vi "dfd_FXP_Expand Filter Quantizers.vi"(11 "FXPOPs":T1[](array[typedef]) {"source" items=["Coef a/k"=0, "Coef b/v"=7, "Input"=1, "Output"=2, "Multiplicand"=3, "Product"=4, "Sum"=5, "Delay"=6, "Gain"=8]}) -> (0 "Delay":T1={"source"=0, "is floating?"=FALSE, "o-mode"=enum."Wrap", "q-mode"=enum."Nearest", "wl"=1, "high limit"=0, "low limit"=0, "iwl"=0, "sign?"=TRUE} {"source" items=["Coef a/k"=0, "Coef b/v"=7, "Input"=1, "Output"=2, "Multiplicand"=3, "Product"=4, "Sum"=5, "Delay"=6, "Gain"=8]}, 1 "Sum":T1={"source"=0, "is floating?"=FALSE, "o-mode"=enum."Wrap", "q-mode"=enum."Nearest", "wl"=1, "high limit"=0, "low limit"=0, "iwl"=0, "sign?"=TRUE} {"source" items=["Coef a/k"=0, "Coef b/v"=7, "Input"=1, "Output"=2, "Multiplicand"=3, "Product"=4, "Sum"=5, "Delay"=6, "Gain"=8]}, 2 "Product":T1={"source"=0, "is floating?"=FALSE, "o-mode"=enum."Wrap", "q-mode"=enum."Nearest", "wl"=1, "high limit"=0, "low limit"=0, "iwl"=0, "sign?"=TRUE} {"source" items=["Coef a/k"=0, "Coef b/v"=7, "Input"=1, "Output"=2, "Multiplicand"=3, "Product"=4, "Sum"=5, "Delay"=6, "Gain"=8]}, 3 "Multiplicand":T1={"source"=0, "is floating?"=FALSE, "o-mode"=enum."Wrap", "q-mode"=enum."Nearest", "wl"=1, "high limit"=0, "low limit"=0, "iwl"=0, "sign?"=TRUE} {"source" items=["Coef a/k"=0, "Coef b/v"=7, "Input"=1, "Output"=2, "Multiplicand"=3, "Product"=4, "Sum"=5, "Delay"=6, "Gain"=8]}, 4 "Coefficient b/v":T1={"source"=0, "is floating?"=FALSE, "o-mode"=enum."Wrap", "q-mode"=enum."Truncation", "wl"=1, "high limit"=0, "low limit"=0, "iwl"=0, "sign?"=TRUE} {"source" items=["Coef a/k"=0, "Coef b/v"=7, "Input"=1, "Output"=2, "Multiplicand"=3, "Product"=4, "Sum"=5, "Delay"=6, "Gain"=8]}, 5 "Output":T1={"source"=0, "is floating?"=FALSE, "o-mode"=enum."Wrap", "q-mode"=enum."Nearest", "wl"=1, "high limit"=0, "low limit"=0, "iwl"=0, "sign?"=TRUE} {"source" items=["Coef a/k"=0, "Coef b/v"=7, "Input"=1, "Output"=2, "Multiplicand"=3, "Product"=4, "Sum"=5, "Delay"=6, "Gain"=8]}, 6 "Coefficient a/k":T1={"source"=0, "is floating?"=FALSE, "o-mode"=enum."Wrap", "q-mode"=enum."Nearest", "wl"=1, "high limit"=0, "low limit"=0, "iwl"=0, "sign?"=TRUE} {"source" items=["Coef a/k"=0, "Coef b/v"=7, "Input"=1, "Output"=2, "Multiplicand"=3, "Product"=4, "Sum"=5, "Delay"=6, "Gain"=8]}, 7 "Input":T1={"source"=0, "is floating?"=FALSE, "o-mode"=enum."Wrap", "q-mode"=enum."Nearest", "wl"=1, "high limit"=0, "low limit"=0, "iwl"=0, "sign?"=TRUE} {"source" items=["Coef a/k"=0, "Coef b/v"=7, "Input"=1, "Output"=2, "Multiplicand"=3, "Product"=4, "Sum"=5, "Delay"=6, "Gain"=8]}, 8 "Gain":T1={"source"=0, "is floating?"=FALSE, "o-mode"=enum."Wrap", "q-mode"=enum."Truncation", "wl"=1, "high limit"=0, "low limit"=0, "iwl"=0, "sign?"=TRUE} {"source" items=["Coef a/k"=0, "Coef b/v"=7, "Input"=1, "Output"=2, "Multiplicand"=3, "Product"=4, "Sum"=5, "Delay"=6, "Gain"=8]})   [LabVIEW 2017, in "NI_DigFilter_FXP.lvlib"]
uses:
  <vilib>/addons/Digital Filter Design/NI_DigFilter_FXP.lvlib
  <vilib>/addons/Digital Filter Design/_Objects.llb/dfd_DFXP Operation Parameter.ctl
  <vilib>/addons/Digital Filter Design/_Objects.llb/dfd_Internal Quantization Srcs.ctl
  <vilib>/addons/Digital Filter Design/NI_DigFilterLicensed.lvlib
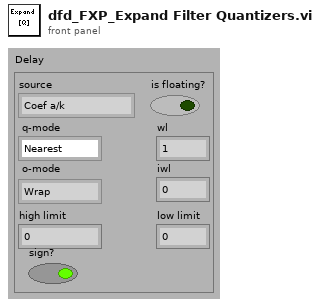
[diagram p1: front panel]
types:
  T1 = typedef "dfd_DFXP Operation Parameter.ctl" = cluster{"source":T2, "is floating?":bool, "o-mode":enum16{"Saturation", "Wrap"}, "q-mode":enum16{"Nearest", "Truncation"}, "wl":i16, "high limit":i64, "low limit":i64, "iwl":i16, "sign?":bool}
  T2 = typedef "NI_DigFilterLicensed.lvlib/dfd_Internal Quantization Srcs.ctl" = u16
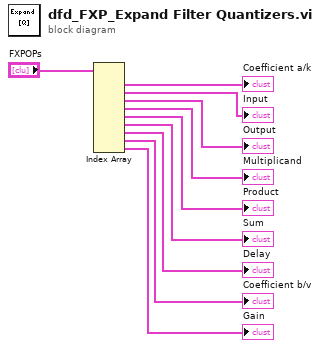
[diagram p0: block diagram]
diagram:
  n1 = Index Array(array="FXPOPs") -> (element #1=→"Coefficient a/k":T1, element #2=→"Input":T1, element #3=→"Output":T1, element #4=→"Multiplicand":T1, element #5=→"Product":T1, element #6=→"Sum":T1, element #7=→"Delay":T1, element #8=→"Coefficient b/v":T1, element #9=→"Gain":T1)  [unwired: 9 in]
